vi "Demo.vi"() -> ()   [LabVIEW 2020, in "BetterDragAndDropDemo.lvlib"]
uses:
  BetterDragAndDropDemo.lvlib
  SubVIs/Horizontal Bar Picture Control.ctl
  SubVIs/EventLoopData.ctl
  Classes/BetterHandle/BetterHandle.lvclass
  Classes/BetterDropOp/BetterDropOp.lvclass
  Demo/Classes/Valve Item/valve color.ctl
  Classes/BetterTreeItem/BetterItem.lvclass/BetterItem.ctl
  Demo/Classes/Folder Item/Folder Item.lvclass
  C:/DSCE code/Open-source/betterdraganddrop_GIT/Source/Classes/BetterTreeItem/BetterItem.lvclass
  Demo/Classes/Valve Item/Valve Item.lvclass
  Classes/BetterTreeHandle/BetterTreeHandle.lvclass
  C:/DSCE code/Open-source/betterdraganddrop_GIT/Source/Classes/BetterHandle/BetterHandle.lvclass
  Classes/BetterMultiListboxHandle/BetterMultiListboxHandle.lvclass
  Classes/BetterListboxHandle/BetterListboxHandle.lvclass
  Classes/BetterMultiListboxHandle/New BetterMultiListboxHandle.vi
  Classes/BetterListboxHandle/New BetterListboxHandle.vi
  Classes/BetterTreeHandle/New BetterTreeHandle.vi
  Classes/BetterTreeItem/BetterItem.lvclass
  Classes/BetterHandle/Add Items (inline).vi
  Classes/BetterHandle/Delete Items (inline).vi
  Classes/BetterHandle/Intra-Move Items (inline).vi
  Classes/BetterHandle/Inter-Move Items (inline).vi
  Classes/BetterHandle/Overwrite Item (inline).vi
  Classes/BetterHandle/New Items (inline).vi
  Classes/BetterHandle/Refresh Item (inline).vi
  Classes/BetterHandle/Drag Over (inline).vi
  Classes/BetterHandle/Drag Leave (inline).vi
  Classes/BetterHandle/Drag Start (inline).vi
  Classes/BetterHandle/Drop (inline).vi
  Classes/BetterHandle/Drag Ended (inline).vi
  Classes/BetterHandle/Valid.vi
  Classes/BetterHandle/Read ItemObjs.vi
  Classes/BetterHandle/Get Ref (inline).vi
  Classes/BetterTreeBar/BetterHorizontalBar.lvclass
panel:
  in  "Scalar Tree":string(tree)
  out "Bar: Scalar Tree":T1
  in  "Array Tree":string[](tree)
  out "Bar: Array Tree":T1
  in  "Scalar MCL":i32(listbox)
  out "Bar: Scalar MCL":T1
  in  "Array MCL":i32[](listbox)
  out "Bar: Array MCL":T1
  in  "Scalar Listbox":i32(listbox)
  out "Bar: Scalar Listbox":T1
  in  "Array Listbox":i32[](listbox)
  out "Bar: Array Listbox":T1
  # "Notes:\n- Use cursor position to change drop indent level when dragging over tree controls\n- Hold \"ctrl\" key to perform \"copy\" when dropping items\n- Drag and drop of multiple items is supported.  (Use ctrl and shift keys to multiselect)\n- All move actions carry children\n- Compatible with Trees, Listboxes, and Multicolumn listboxes\n- Compatible with either \"scalar\" or \"array\" datatype of afformentioned controls\n- Only the \"folder\" item below allows children.  This is a method of the item."
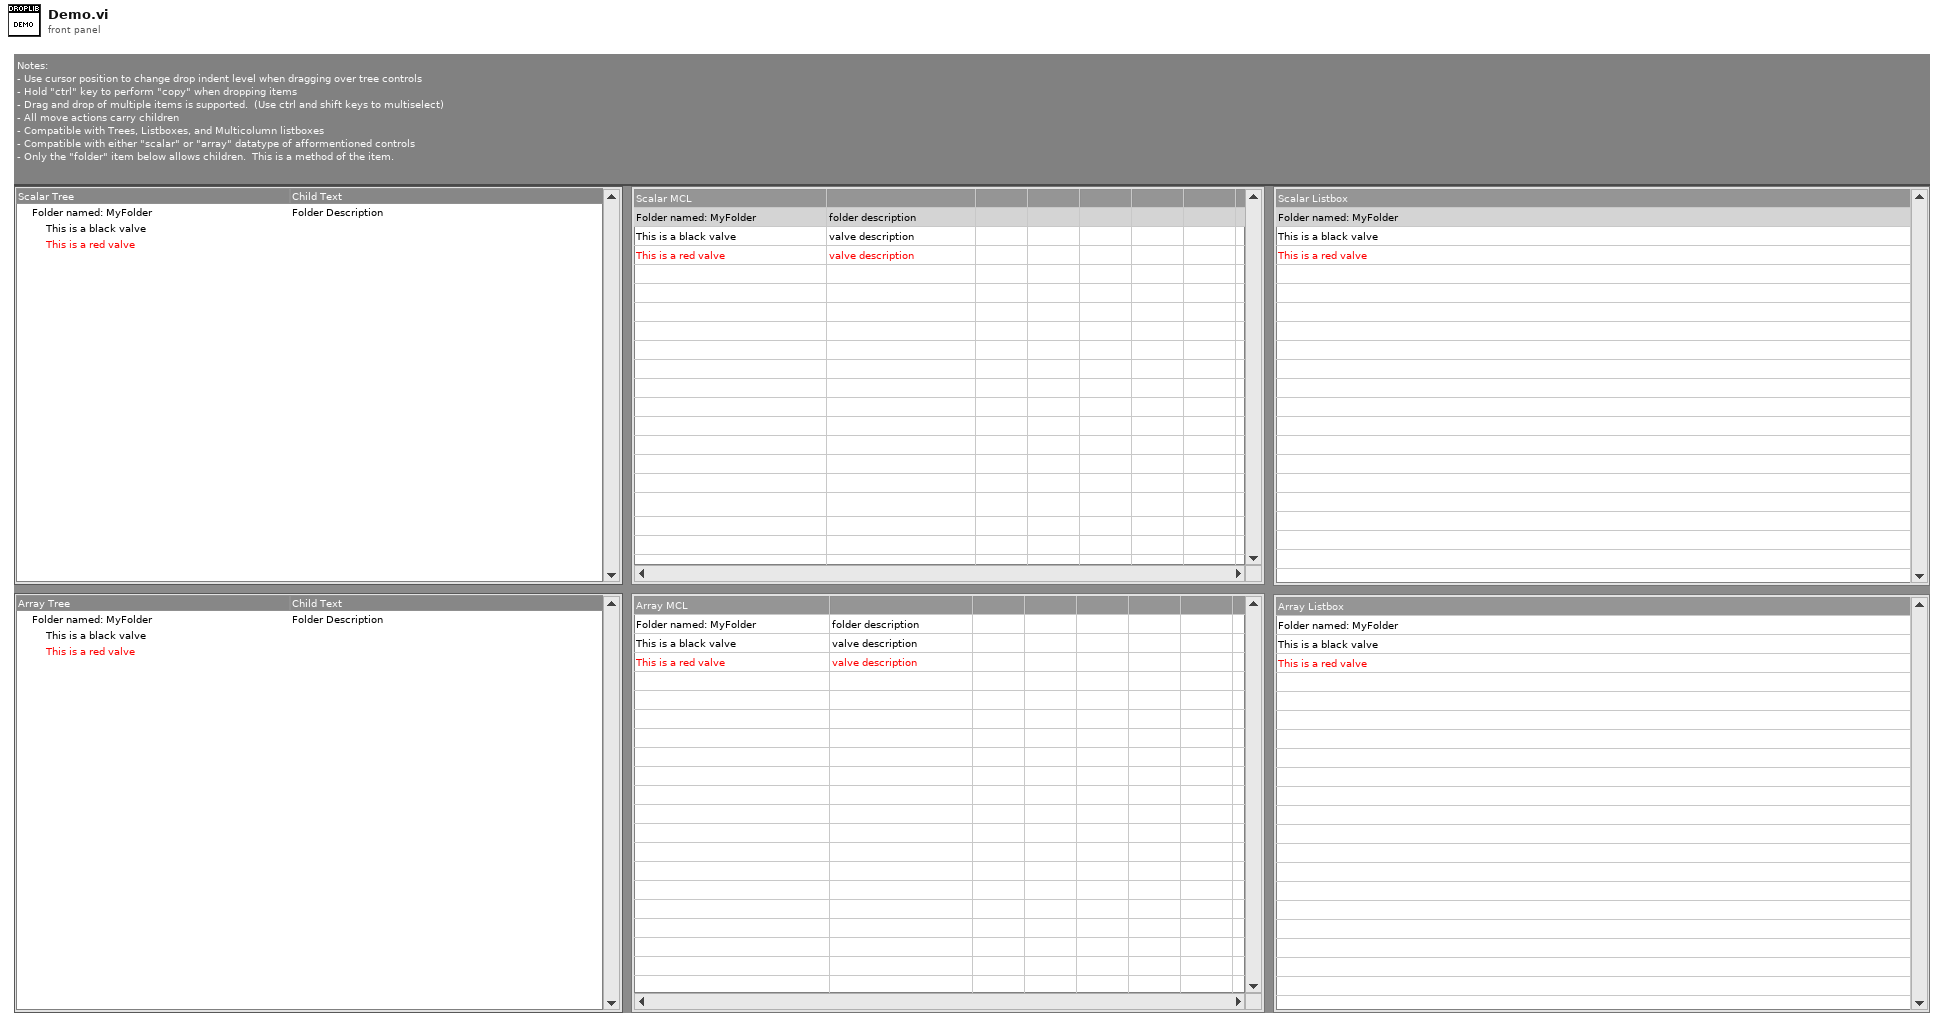
[diagram p1: front panel]
types:
  T1 = typedef "BetterDragAndDrop.lvlib/BetterHorizontalBar.lvclass/Horizontal Bar Picture Control.ctl" = picture
  T2 = typedef "BetterDragAndDropDemo.lvlib/Valve Item.lvclass/valve color.ctl" = enum16{"black", "red"}
  T3 = typedef "BetterDragAndDropDemo.lvlib/EventLoopData.ctl" = cluster{"Handles":refnum<class "BetterHandle.lvclass">[], "BetterDropOp":refnum<class "BetterDropOp.lvclass">}
  T4 = typedef "LVPoint32TypeDef.ctl" = cluster{"Horizontal":i32, "Vertical":i32}
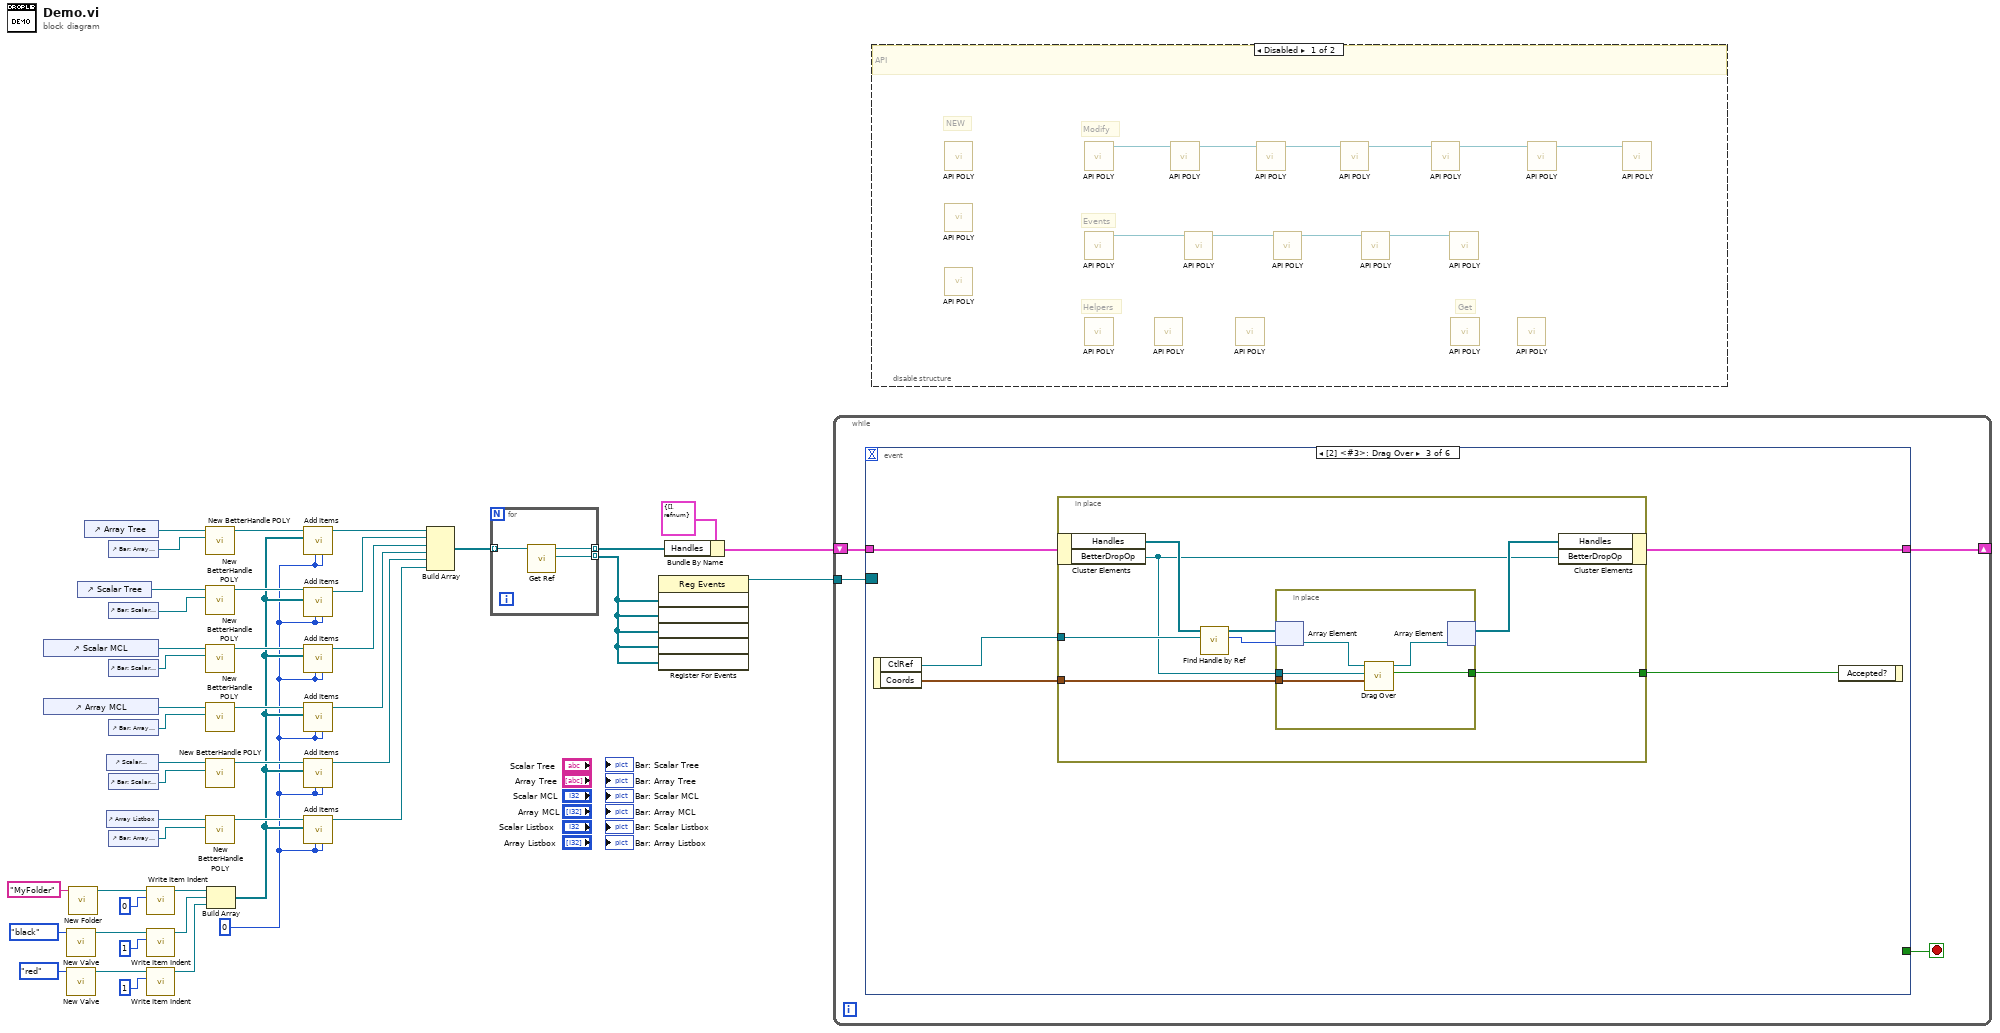
[diagram p0: block diagram]
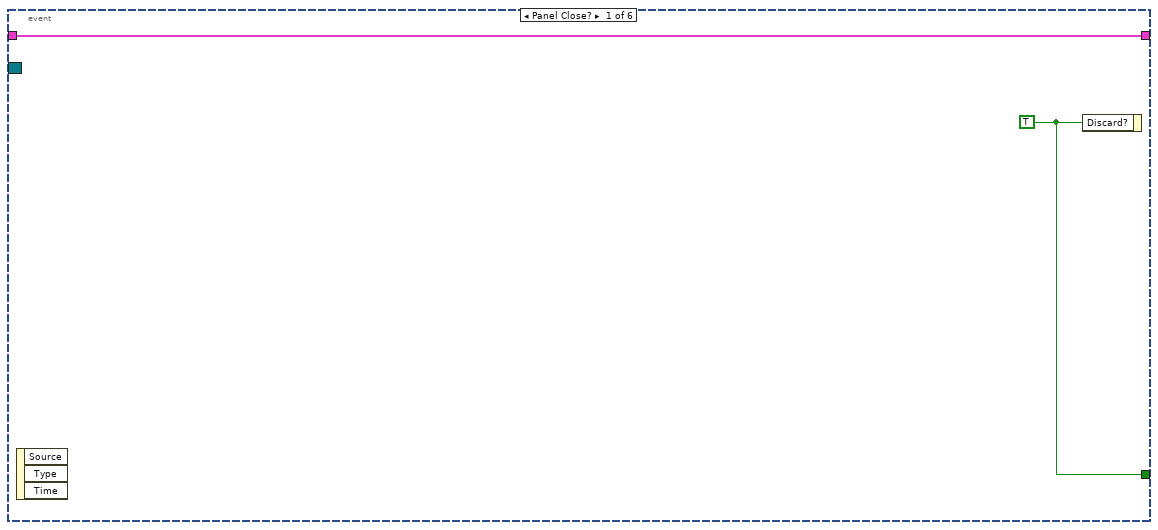
[diagram p3: hidden frame]
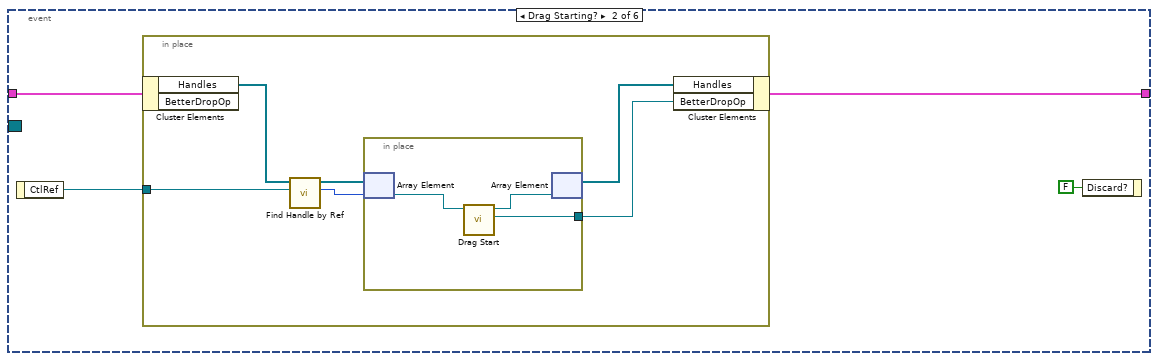
[diagram p4: hidden frame]
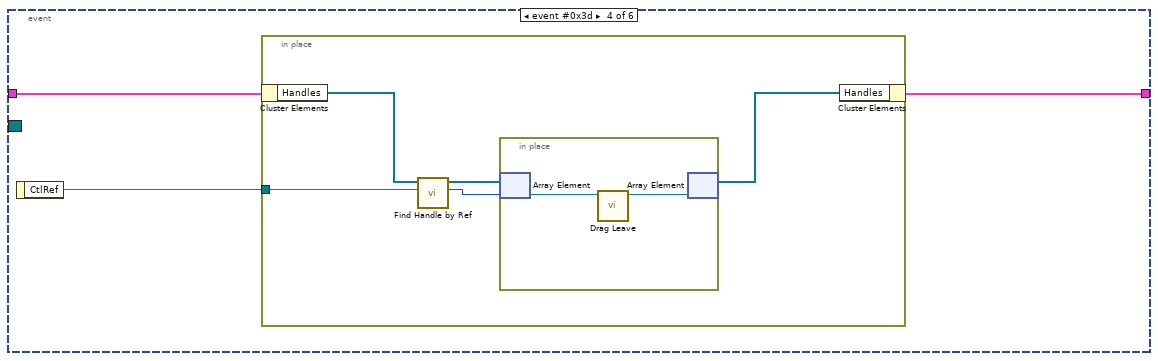
[diagram p5: hidden frame]
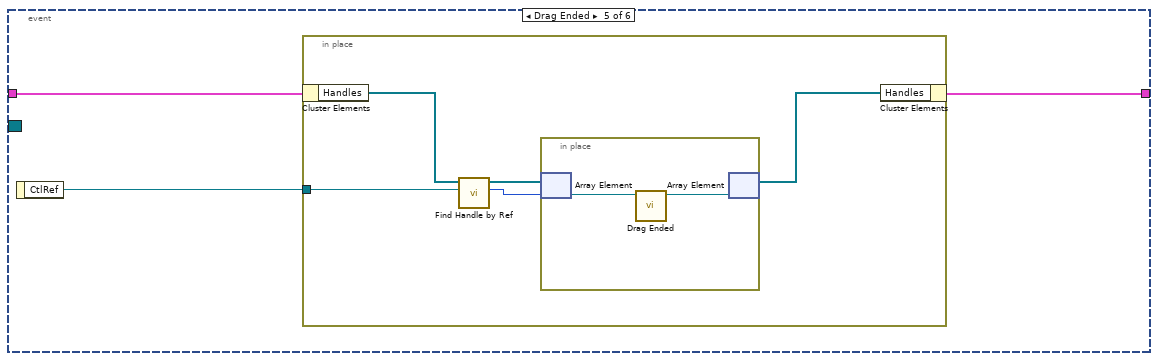
[diagram p6: hidden frame]
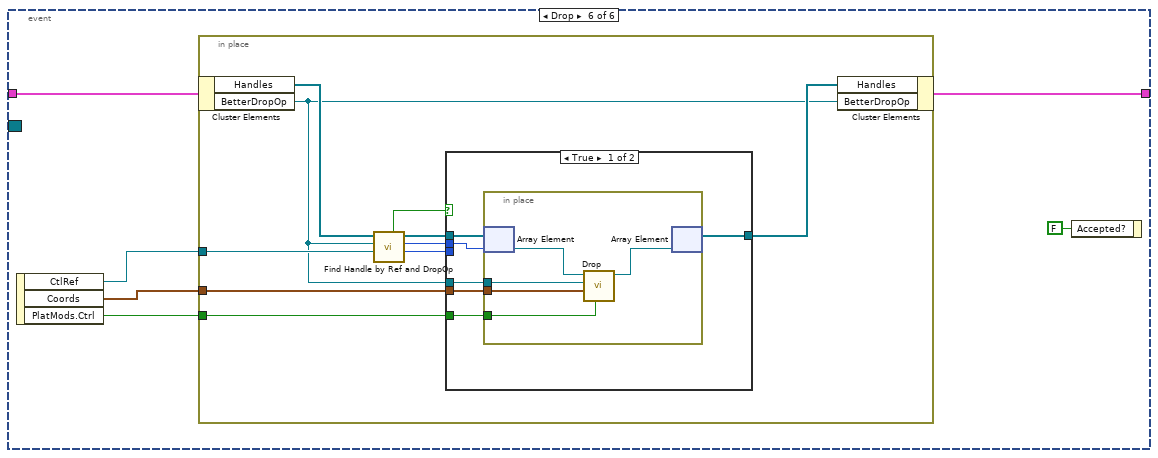
[diagram p7: hidden frame]
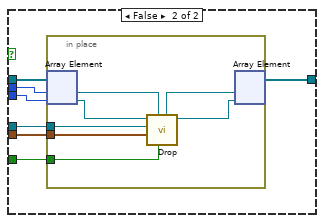
[diagram p8: hidden frame]
diagram:
  w5 = 0 ("Insertion index")
  n1 = control-ref of="Scalar MCL"() -> (w41:refnum<vi>)
  n2 = control-ref of="Array MCL"() -> (w40:refnum<vi>)
  n3 = call "New Valve.vi"("valve color"=valve_color."black") -> ("Valve Item out"=w25:refnum<class "Valve Item.lvclass">)  [unwired: 9 in, 1 out]
  n4 = call "New Valve.vi"("valve color"=valve_color."red") -> ("Valve Item out"=w23:refnum<class "Valve Item.lvclass">)  [unwired: 9 in, 1 out]
  n5 = call "New Folder.vi"("folder name"="MyFolder") -> ("Folder Item out"=w28:refnum<class "Folder Item.lvclass">)  [unwired: 9 in, 1 out]
  n6 = control-ref of="Scalar Tree"() -> (w11:refnum<vi>)
  n7 = control-ref of="Array Tree"() -> (w12:refnum<vi>)
  n8 = control-ref of="Scalar Listbox"() -> (w39:refnum<vi>)
  n9 = control-ref of="Array Listbox"() -> (w38:refnum<vi>)
  n10 = control-ref of="Bar: Array Tree"() -> (w17:refnum<vi>)
  n11 = control-ref of="Bar: Scalar Tree"() -> (w18:refnum<vi>)
  n12 = control-ref of="Bar: Scalar MCL"() -> (w37:refnum<vi>)
  n13 = control-ref of="Bar: Array MCL"() -> (w36:refnum<vi>)
  n14 = control-ref of="Bar: Scalar Listbox"() -> (w35:refnum<vi>)
  n15 = control-ref of="Bar: Array Listbox"() -> (w34:refnum<vi>)
  n16 = call "Write Item Indent.vi"("Item Indent"=0, "BetterTreeItem in"=w28) -> ("BetterTreeItem out"=w22:refnum<class "Folder Item.lvclass">)  [unwired: 9 in]
  n17 = call "Write Item Indent.vi"("Item Indent"=1, "BetterTreeItem in"=w25) -> ("BetterTreeItem out"=w21:refnum<class "Valve Item.lvclass">)  [unwired: 9 in]
  n18 = call "Write Item Indent.vi"("Item Indent"=1, "BetterTreeItem in"=w23) -> ("BetterTreeItem out"=w20:refnum<class "Valve Item.lvclass">)  [unwired: 9 in]
  n19 = call-poly "New BetterHandle POLY.vi"("TreeBar Picture Ref"=w17, "TreeRef"=w12) -> ("BetterTreeHandle out"=w16:refnum<class "BetterTreeHandle.lvclass">)  [unwired: 8 in, 1 out]
  n20 = call-poly "New BetterHandle POLY.vi"("TreeBar Picture Ref"=w18, "TreeRef"=w11) -> ("BetterTreeHandle out"=w14:refnum<class "BetterTreeHandle.lvclass">)  [unwired: 8 in, 1 out]
  n21 = call-poly "New BetterHandle POLY.vi"("TreeBar Picture Ref"=w37, "MCL ref"=w41) -> ("BetterMultiListboxHandle out"=w10:refnum<class "BetterMultiListboxHandle.lvclass">)  [unwired: 8 in, 1 out]
  n22 = call-poly "New BetterHandle POLY.vi"("TreeBar Picture Ref"=w36, "MCL ref"=w40) -> ("BetterMultiListboxHandle out"=w9:refnum<class "BetterMultiListboxHandle.lvclass">)  [unwired: 8 in, 1 out]
  n23 = call-poly "New BetterHandle POLY.vi"("TreeBar Picture Ref"=w35, "LB ref"=w39) -> ("BetterListboxHandle out"=w8:refnum<class "BetterListboxHandle.lvclass">)  [unwired: 8 in, 1 out]
  n24 = call-poly "New BetterHandle POLY.vi"("TreeBar Picture Ref"=w34, "LB ref"=w38) -> ("BetterListboxHandle out"=w7:refnum<class "BetterListboxHandle.lvclass">)  [unwired: 8 in, 1 out]
  n25 = Build Array(w22, w21, w20) -> (w6:refnum<class "BetterItem.lvclass">[])
  n26 = call-dynamic "Add Items.vi"("indent"=w5, "Insertion index"=w5, "Items to Add"=w6, "Better Tree Handle In"=w16) -> ("Better Tree Handle Out"=w19:refnum<class "BetterTreeHandle.lvclass">)  [unwired: 6 in, 1 out]
  n27 = call-dynamic "Add Items.vi"("indent"=w5, "Insertion index"=w5, "Items to Add"=w6, "Better Tree Handle In"=w14) -> ("Better Tree Handle Out"=w13:refnum<class "BetterTreeHandle.lvclass">)  [unwired: 6 in, 1 out]
  n28 = call-dynamic "Add Items.vi"("indent"=w5, "Insertion index"=w5, "Items to Add"=w6, "BetterBoxHandle in"=w10) -> ("BetterBoxHandle out"=w4:refnum<class "BetterMultiListboxHandle.lvclass">)  [unwired: 6 in, 1 out]
  n29 = call-dynamic "Add Items.vi"("indent"=w5, "Insertion index"=w5, "Items to Add"=w6, "BetterBoxHandle in"=w9) -> ("BetterBoxHandle out"=w3:refnum<class "BetterMultiListboxHandle.lvclass">)  [unwired: 6 in, 1 out]
  n30 = call-dynamic "Add Items.vi"("indent"=w5, "Insertion index"=w5, "Items to Add"=w6, "BetterBoxHandle in"=w8) -> ("BetterBoxHandle out"=w2:refnum<class "BetterListboxHandle.lvclass">)  [unwired: 6 in, 1 out]
  n31 = call-dynamic "Add Items.vi"("indent"=w5, "Insertion index"=w5, "Items to Add"=w6, "BetterBoxHandle in"=w7) -> ("BetterBoxHandle out"=w1:refnum<class "BetterListboxHandle.lvclass">)  [unwired: 6 in, 1 out]
  n32 = Build Array(w19, w13, w4, w3, w2, w1) -> (w33:refnum<class "BetterHandle.lvclass">[])
  n33 = for {
    tunnel: w33 -> [w47] mode=indexing
    tunnel: [w46] -> w32 mode=indexing
    tunnel: [w45] -> w15 mode=indexing
    n34 = call-dynamic "Get Ref.vi"("BetterHandle in"=w47) -> ("Tree/LB/MCL ref"=w45:refnum<vi>, "BetterHandle out"=w46:refnum<class "BetterHandle.lvclass">)  [unwired: 8 in, 1 out]
  }
  n35 = register-events(w15, w15, w15, w15, w15) -> (reference out=w43:refnum<event-registration>)  [unwired: 2 in, 1 out]
  n36 = Bundle By Name(cluster=T3 {"Handles"=[], "BetterDropOp"=refnum} ("Cluster 2"), "Handles"=w32) -> (w44:T3)
  n37 = while {
    shift-right: [w49] -> _
    shift-left: w44 -> [w50]
    tunnel: w43 -> [w48]
    stop <- w51 stop-if-true
    n38 = event shown="[2] <#3>: Drag Over" {
      selector: w48 -> [_ _ _ _ _ _]
      dyn-events: _ -> [_ _ _ _ _ _]
      timeout: _ -> [_ _ _ _ _ _]
      tunnel: [w52 _ _ _ _ _] -> w51
      tunnel: w50 -> [w53 w57 w71 w87 w97 w110]
      tunnel: [w53 w56 w70 w86 w96 w105] -> w49
      event Panel Close? {
        w52 = TRUE ("Discard?")
        n39 = event-data() -> ()  [unwired: 1 in, 3 out]
        n40 = event-data("Discard?"=w52) -> ()  [unwired: 1 in, 1 out]
      }
      event Drag Starting? {
        n41 = event-data() -> ("CtlRef"=w55:refnum<vi>)  [unwired: 1 in]
        n42 = in-place {
          in-place-border: w55 -> [w58]
          n43 = in-place-cluster #1(w57) -> ("Handles"=w63:refnum<class "BetterHandle.lvclass">[])  [unwired: 1 out]
          n44 = call "Find Handle by Ref.vi"("Ref"=w58, "BetterHandle array"=w63) -> ("Handle index"=w61:i32, "BetterHandle array"=w62:refnum<class "BetterHandle.lvclass">[])  [unwired: 7 in, 1 out]
          n45 = in-place {
            in-place-border: [w64] -> w59
            n46 = in-place-array #2(w62, w61) -> (w66:refnum<class "BetterHandle.lvclass">)
            n47 = call-dynamic "Drag Start.vi"("BetterHandle in"=w66) -> ("BetterDropOp"=w64:refnum<class "BetterDropOp.lvclass">, "BetterHandle out"=w65:refnum<class "BetterHandle.lvclass">)  [unwired: 8 in, 1 out]
            n48 = in-place-array #2(w65) -> (w60:refnum<class "BetterHandle.lvclass">[])  [unwired: 1 out]
          }
          n49 = in-place-cluster #1("Handles"=w60, "BetterDropOp"=w59) -> (w56:T3)
        }
        n50 = event-data("Discard?"=FALSE) -> ()  [unwired: 1 in, 1 out]
      }
      event event type 1.0.xa000003a {
        n51 = event-data() -> ("CtlRef"=w69:refnum<vi>, "Coords"=w68:T4)  [unwired: 1 in]
        n52 = in-place {
          in-place-border: w69 -> [w75]
          in-place-border: w68 -> [w73]
          in-place-border: [w72] -> w67
          n53 = in-place-cluster #3(w71) -> ("Handles"=w79:refnum<class "BetterHandle.lvclass">[], "BetterDropOp"=w74:refnum<class "BetterDropOp.lvclass">)
          n54 = call "Find Handle by Ref.vi"("Ref"=w75, "BetterHandle array"=w79) -> ("Handle index"=w77:i32, "BetterHandle array"=w78:refnum<class "BetterHandle.lvclass">[])  [unwired: 7 in, 1 out]
          n55 = in-place {
            in-place-border: w74 -> [w82]
            in-place-border: w73 -> [w81]
            in-place-border: [w80] -> w72
            n56 = in-place-array #4(w78, w77) -> (w84:refnum<class "BetterHandle.lvclass">)
            n57 = call "Drag Over.vi"("Coords"=w81, "BetterDropOp"=w82, "BetterHandle in"=w84) -> ("Drag Accepted?"=w80:bool, "BetterHandle out"=w83:refnum<class "BetterHandle.lvclass">)  [unwired: 6 in, 1 out]
            n58 = in-place-array #4(w83) -> (w76:refnum<class "BetterHandle.lvclass">[])  [unwired: 1 out]
          }
          n59 = in-place-cluster #3("Handles"=w76, "BetterDropOp"=w74) -> (w70:T3)
        }
        n60 = event-data("Accepted?"=w67) -> ()  [unwired: 1 in, 1 out]
      }
      event event #0x3d {
        n61 = event-data() -> ("CtlRef"=w85:refnum<vi>)  [unwired: 1 in]
        n62 = in-place {
          in-place-border: w85 -> [w88]
          n63 = in-place-cluster #5(w87) -> ("Handles"=w92:refnum<class "BetterHandle.lvclass">[])
          n64 = call "Find Handle by Ref.vi"("Ref"=w88, "BetterHandle array"=w92) -> ("Handle index"=w90:i32, "BetterHandle array"=w91:refnum<class "BetterHandle.lvclass">[])  [unwired: 7 in, 1 out]
          n65 = in-place {
            n66 = in-place-array #6(w91, w90) -> (w94:refnum<class "BetterHandle.lvclass">)
            n67 = call-dynamic "Drag Leave.vi"("BetterHandle in"=w94) -> ("BetterHandle out"=w93:refnum<class "BetterHandle.lvclass">)  [unwired: 9 in, 1 out]
            n68 = in-place-array #6(w93) -> (w89:refnum<class "BetterHandle.lvclass">[])  [unwired: 1 out]
          }
          n69 = in-place-cluster #5("Handles"=w89) -> (w86:T3)
        }
      }
      event Drag Ended {
        n70 = event-data() -> ("CtlRef"=w95:refnum<vi>)  [unwired: 1 in]
        n71 = in-place {
          in-place-border: w95 -> [w98]
          n72 = in-place-cluster #7(w97) -> ("Handles"=w102:refnum<class "BetterHandle.lvclass">[])
          n73 = call "Find Handle by Ref.vi"("Ref"=w98, "BetterHandle array"=w102) -> ("Handle index"=w100:i32, "BetterHandle array"=w101:refnum<class "BetterHandle.lvclass">[])  [unwired: 7 in, 1 out]
          n74 = in-place {
            n75 = in-place-array #8(w101, w100) -> (w104:refnum<class "BetterHandle.lvclass">)
            n76 = call-dynamic "Drag Ended.vi"("BetterHandle in"=w104) -> ("BetterHandle out"=w103:refnum<class "BetterHandle.lvclass">)  [unwired: 9 in, 1 out]
            n77 = in-place-array #8(w103) -> (w99:refnum<class "BetterHandle.lvclass">[])  [unwired: 1 out]
          }
          n78 = in-place-cluster #7("Handles"=w99) -> (w96:T3)
        }
      }
      event Drop {
        n79 = event-data() -> ("CtlRef"=w109:refnum<vi>, "Coords"=w108:T4, "PlatMods.Ctrl"=w106:bool)  [unwired: 1 in]
        n80 = in-place {
          in-place-border: w109 -> [w118]
          in-place-border: w108 -> [w116]
          in-place-border: w106 -> [w114]
          n81 = in-place-cluster #9(w110) -> ("Handles"=w119:refnum<class "BetterHandle.lvclass">[], "BetterDropOp"=w115:refnum<class "BetterDropOp.lvclass">)
          n82 = call "Find Handle by Ref and DropOp.vi"("Ref (Destination)"=w118, "BetterDropOp (Source)"=w115, "BetterHandle array"=w119) -> ("Handle index (Destination)"=w111:i32, "Handle index (Source)"=w112:i32, "BetterHandle array"=w117:refnum<class "BetterHandle.lvclass">[], "Source and Destination are the same?"=w113:bool)  [unwired: 4 in, 1 out]
          n83 = case shown="True" w113 {
            tunnel: [w126 w138] -> w120
            tunnel: w117 -> [w125 w137]
            tunnel: w116 -> [w124 w136]
            tunnel: w115 -> [w123 w135]
            tunnel: w114 -> [w122 w134]
            tunnel: w112 -> [w121 w133]
            tunnel: w111 -> [_ w132]
            frame True {
              n84 = in-place {
                in-place-border: w124 -> [w129]
                in-place-border: w123 -> [w130]
                in-place-border: w122 -> [w128]
                n85 = in-place-array #10(w125, w121) -> (w127:refnum<class "BetterHandle.lvclass">)
                n86 = call "Drop.vi"("Copy?"=w128, "Coords"=w129, "BetterDropOp"=w130, "BetterHandle in (destination)"=w127) -> ("BetterHandle out (destination)"=w131:refnum<class "BetterHandle.lvclass">)  [unwired: 5 in, 2 out]
                n87 = in-place-array #10(w131) -> (w126:refnum<class "BetterHandle.lvclass">[])  [unwired: 1 out]
              }
            }
            frame False {
              n88 = in-place {
                in-place-border: w136 -> [w144]
                in-place-border: w135 -> [w145]
                in-place-border: w134 -> [w143]
                n89 = in-place-array #11(w137, w133, w132) -> (w142:refnum<class "BetterHandle.lvclass">, w139:refnum<class "BetterHandle.lvclass">)
                n90 = call "Drop.vi"("Copy?"=w143, "BetterHandle in (source)"=w142, "Coords"=w144, "BetterDropOp"=w145, "BetterHandle in (destination)"=w139) -> ("BetterHandle out (destination)"=w140:refnum<class "BetterHandle.lvclass">, "BetterHandle out (source)"=w141:refnum<class "BetterHandle.lvclass">)  [unwired: 4 in, 1 out]
                n91 = in-place-array #11(w141, w140) -> (w138:refnum<class "BetterHandle.lvclass">[])  [unwired: 2 out]
              }
            }
          }
          n92 = in-place-cluster #9("Handles"=w120, "BetterDropOp"=w115) -> (w105:T3)
        }
        n93 = event-data("Accepted?"=FALSE) -> ()  [unwired: 1 in, 1 out]
      }
    }
  }
  n94 = disable-structure shown="Disabled" {
    frame Disabled {
      # "Get"
      # "Helpers"
      # "Events"
      # "Modify"
      # "NEW"
      # "API"
      n95 = call-poly "API POLY.vi"() -> ()  [unwired: 10 in, 2 out]
      n96 = call-poly "API POLY.vi"() -> ()  [unwired: 10 in, 2 out]
      n97 = call-poly "API POLY.vi"() -> ()  [unwired: 10 in, 2 out]
      n98 = call-poly "API POLY.vi"() -> ("BetterHandle out"=w146:refnum<class "BetterHandle.lvclass">)  [unwired: 10 in, 1 out]
      n99 = call-poly "API POLY.vi"() -> ("BetterHandle out"=w150:refnum<class "BetterHandle.lvclass">)  [unwired: 9 in, 2 out]
      n100 = call-poly "API POLY.vi"() -> ()  [unwired: 9 in, 3 out]
      n101 = call-poly "API POLY.vi"() -> ()  [unwired: 9 in, 3 out]
      n102 = call-poly "API POLY.vi"("BetterHandle in"=w146) -> ("BetterHandle out"=w155:refnum<class "BetterHandle.lvclass">)  [unwired: 8 in, 2 out]
      n103 = call-poly "API POLY.vi"("BetterHandle in"=w150) -> ("BetterHandle out"=w149:refnum<class "BetterHandle.lvclass">)  [unwired: 8 in, 2 out]
      n104 = call-poly "API POLY.vi"() -> ()  [unwired: 7 in, 5 out]
      n105 = call-poly "API POLY.vi"("BetterHandle in"=w155) -> ("BetterHandle out"=w154:refnum<class "BetterHandle.lvclass">)  [unwired: 9 in, 1 out]
      n106 = call-poly "API POLY.vi"("BetterHandle in"=w149) -> ("BetterHandle out"=w148:refnum<class "BetterHandle.lvclass">)  [unwired: 9 in, 1 out]
      n107 = call-poly "API POLY.vi"("BetterHandle in (destination)"=w154) -> ("BetterHandle out (destination)"=w153:refnum<class "BetterHandle.lvclass">)  [unwired: 8 in, 2 out]
      n108 = call-poly "API POLY.vi"("BetterHandle in (destination)"=w148) -> ("BetterHandle out (destination)"=w147:refnum<class "BetterHandle.lvclass">)  [unwired: 8 in, 2 out]
      n109 = call-poly "API POLY.vi"("BetterHandle in"=w153) -> ("BetterHandle out"=w152:refnum<class "BetterHandle.lvclass">)  [unwired: 9 in, 1 out]
      n110 = call-poly "API POLY.vi"("BetterHandle in"=w147) -> ()  [unwired: 9 in, 2 out]
      n111 = call-poly "API POLY.vi"() -> ()  [unwired: 10 in, 2 out]
      n112 = call-poly "API POLY.vi"() -> ()  [unwired: 9 in, 3 out]
      n113 = call-poly "API POLY.vi"("BetterHandle in"=w152) -> ("BetterHandle out"=w151:refnum<class "BetterHandle.lvclass">)  [unwired: 9 in, 1 out]
      n114 = call-poly "API POLY.vi"("BetterHandle in"=w151) -> ()  [unwired: 9 in, 2 out]
    }
    frame Enabled {
    }
  }
